vi "file -- list data files in mmddyy folder.vi"(11 "<mmddyy> folder path":path) -> (1 "Array":T1(array[cluster]))   [LabVIEW 2010]
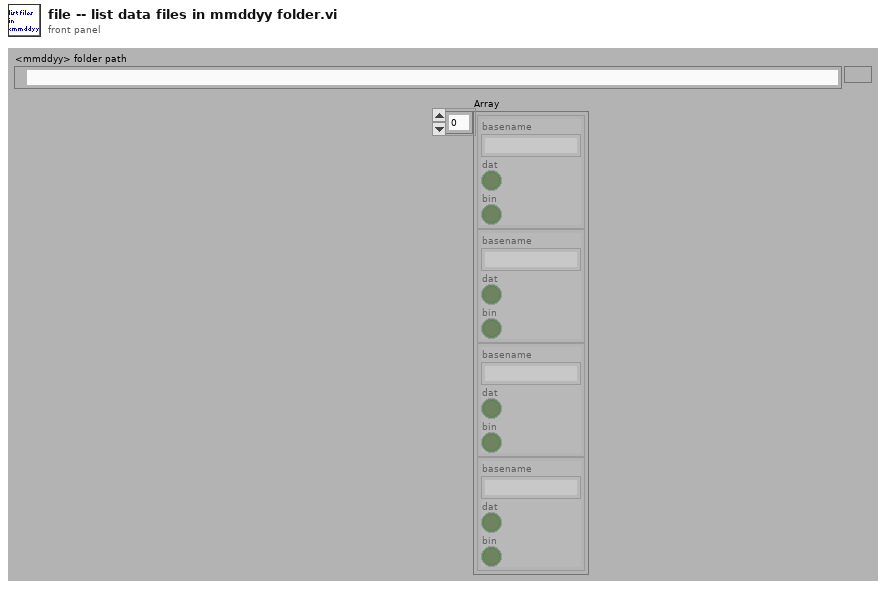
[diagram p1: front panel]
types:
  T1 = cluster{"basename":string, "dat":bool, "bin":bool}[]
  T2 = cluster{"basename":string, "dat":bool, "bin":bool}
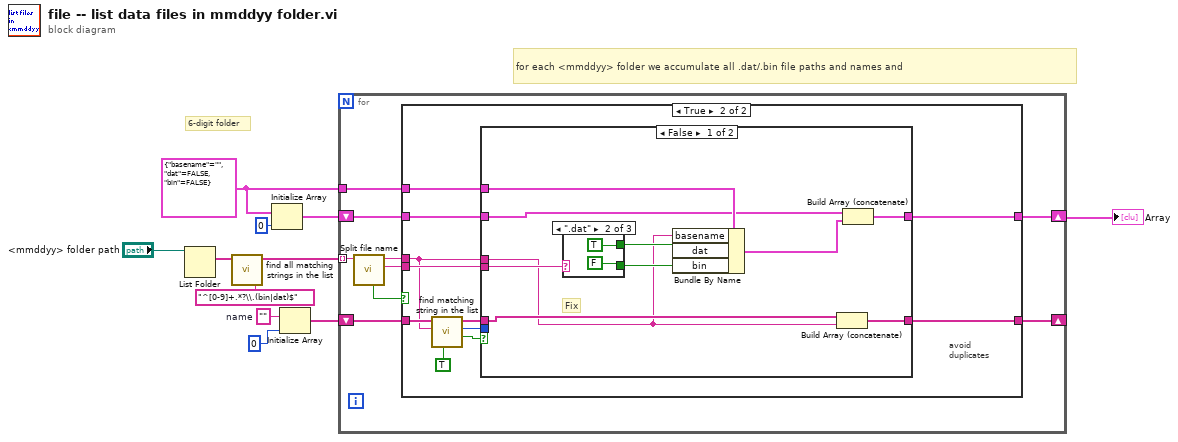
[diagram p0: block diagram]
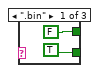
[diagram p3: hidden frame]
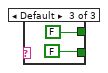
[diagram p4: hidden frame]
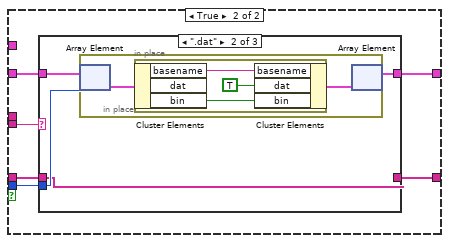
[diagram p5: hidden frame]
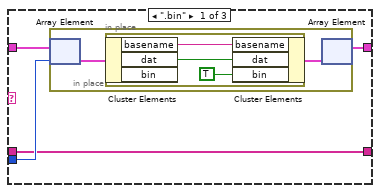
[diagram p6: hidden frame]
diagram:
  w2 = T2 {"basename"="", "dat"=FALSE, "bin"=FALSE}
  w6 = ""  # name
  # "6-digit folder"
  # "for each <mmddyy> folder we accumulate all .dat/.bin file paths and names and"
  n1 = List Folder(path="<mmddyy> folder path") -> (filenames=w11:string[])  [unwired: 3 in, 3 out]
  n2 = call "find all matching strings in the list.vi"("regular expression"="^[0-9]+.*?\\.(bin|dat)$" ("pattern"), "strings"=w11) -> ("list of matching strings"=w9:string[])  [unwired: 7 in, 2 out]
  n3 = Initialize Array(w2, 0) -> (w4:T1)
  n4 = Initialize Array(w6, 0) -> (w5:string[])
  n5 = for {
    tunnel: w9 -> [w20] mode=indexing
    shift-right: [w16] -> _
    shift-left: w5 -> [w15]
    shift-right: [w17] -> w3
    shift-left: w4 -> [w19]
    tunnel: w2 -> [w14]
    n6 = call "Split file name.vi"("file name"=w20) -> ("extension"=w18:string, "name"=w13:string, "exact match"=w12:bool)  [unwired: 8 in]
    n7 = case shown="True" w12 {
      tunnel: w19 -> [w22 w30]
      tunnel: w18 -> [_ w29]
      tunnel: [w22 w27] -> w17
      tunnel: [w21 w26] -> w16
      tunnel: w15 -> [w21 w25]
      tunnel: w14 -> [_ w24]
      tunnel: w13 -> [_ w23]
      frame False {
      }
      frame True {
        # "avoid \nduplicates"
        n8 = call "find matching string in the list.vi"("quote specials"=TRUE, "regular expression"=w23, "strings"=w25) -> ("match found"=w31:bool, "matching string index"=w28:i32)  [unwired: 6 in, 1 out]
        n9 = case shown="False" w31 {
          tunnel: w30 -> [w36 w54]
          tunnel: w29 -> [w39 w53]
          tunnel: w28 -> [_ w52]
          tunnel: [w34 w51] -> w27
          tunnel: [w41 w50] -> w26
          tunnel: w25 -> [w42 w49]
          tunnel: w23 -> [w33 _]
          tunnel: w24 -> [w40 _]
          frame False {
            # "Fix"
            n10 = case shown="\".dat\"" w39 {
              tunnel: [FALSE ("quote specials") TRUE ("quote specials") FALSE ("quote specials")] -> w38
              tunnel: [TRUE ("quote specials") FALSE ("quote specials") FALSE ("quote specials")] -> w37
              frame ".bin" {
              }
              frame ".dat" {
              }
              frame Default {
              }
            }
            n11 = Bundle By Name(cluster=w40, "basename"=w33, "dat"=w38, "bin"=w37) -> (w35:T2)
            n12 = Build Array (concatenate)(w42, w33) -> (w41:string[])
            n13 = Build Array (concatenate)(w36, w35) -> (w34:T1)
          }
          frame True {
            n14 = case shown="\".dat\"" w53 {
              tunnel: w54 -> [w58 w67 w74]
              tunnel: w52 -> [w56 w66 _]
              tunnel: [w57 w65 w74] -> w51
              tunnel: [w55 w64 w73] -> w50
              tunnel: w49 -> [w55 w64 w73]
              frame ".bin" {
                n15 = in-place {
                  n16 = in-place-array #1(w58, w56) -> (w60:T2)
                  n17 = in-place {
                    n18 = in-place-cluster #2(w60) -> ("basename"=w63:string, "dat"=w61:bool)  [unwired: 1 out]
                    n19 = in-place-cluster #2("basename"=w63, "dat"=w61, "bin"=TRUE ("quote specials")) -> (w59:T2)
                  }
                  n20 = in-place-array #1(w59) -> (w57:T1)  [unwired: 1 out]
                }
              }
              frame ".dat" {
                n21 = in-place {
                  n22 = in-place-array #3(w67, w66) -> (w69:T2)
                  n23 = in-place {
                    n24 = in-place-cluster #4(w69) -> ("basename"=w72:string, "bin"=w71:bool)  [unwired: 1 out]
                    n25 = in-place-cluster #4("basename"=w72, "dat"=TRUE ("quote specials"), "bin"=w71) -> (w68:T2)
                  }
                  n26 = in-place-array #3(w68) -> (w65:T1)  [unwired: 1 out]
                }
              }
              frame Default {
                # "should not get here"
              }
            }
          }
        }
      }
    }
  }
  "Array" <- w3
